vi "Read Config.vi"() -> ()   [LabVIEW 2018]
uses:
  File Type.ctl
  Type Defs/Global Action.ctl
  GC-MSMSDevlopment/Type/_RT Configuration 2.ctl
  Type Defs/Configration.ctl
panel:
  out "Cal/Res":dbl[][](array[numeric])
  out "Configration":T1
  out "Error Out":errorcluster
  in  "Error In":errorcluster
  in  "Start Path":path
  in  "Display (T)":bool=TRUE
  in  "Config File Type":T3
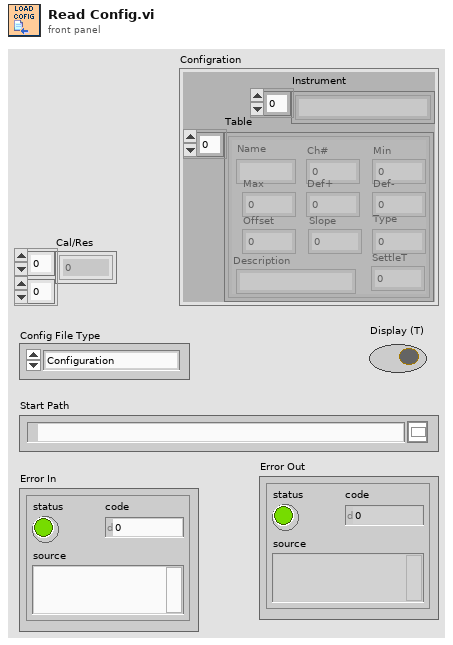
[diagram p1: front panel]
types:
  T1 = typedef "Configration.ctl" = cluster{"Table":T2[], "Instrument":string[]}
  T2 = typedef "_RT Configuration 2.ctl" = cluster{"Name":string, "Ch#":u8, "Min":dbl, "Max":dbl, "Def+":dbl, "Def-":dbl, "Offset":dbl, "Slope":dbl, "Type":u8, "Description":string, "SettleT":dbl}
  T3 = typedef "File Type.ctl" = enum16{"Configuration", "Old Configuration", "Calibration", "Resolution", "Diagnostic Method", "Old Method", "Acq Method", "Samp List"}
  T4 = typedef "Global Action.ctl" = enum16{"Write", "Read"}
  T5 = typedef "Global Configrations.ctl" = cluster{"Model Name":enum16{"QSight 110", "QSight 120", "QSight 210", "QSight 220", "QSight 410", "QSight 420", "IONICS 3Q 110", "IONICS 3Q 120", "IONICS 3Q 210", "IONICS 3Q 220", "IONICS 3Q 310", "IONICS 3Q 320", "Simulation (Single Source)", "Simulation (Dual Source)"}, "RunType":u16, "Acquisition State":enum16{"Ready", "Busy", "Waiting"}, "InstrState":enum16{"Initializing", "Mass Spectrometer is Off", "Starting Up", "Turning Power Off", "Going to Standby", "Roughing Pump Ready", "Turning Turbo Off", "Turbo Startup", "Turbopump Ready", "Checking Vacuum", "Going to Ready", "Ready", "Running", "Source Standby", "Lost Communication", "Shutting Down", "Fault", "24V Standby", "Go to 24V Standby", "Turbopump Ready-Waiting"}, "Run Mode":enum16{"MRM (Q1/Q2)", "Q1 Scan", "Q1 SRM", "Q2 Scan", "Q2 SRM", "Product Scan", "Precursor Scan", "Neutral Loss", "Neutral Gain"}, "Configration":T1, "TCP ID":refnum<k5>, "DT":bool, "Dead Time (nS)":i32, "Single Source":bool, "ADC Tables":T6[], "FW Udate":bool, "Simulator":bool}
  T6 = typedef "ADC Table.ctl" = cluster{"Name":string, "Ch#":u8, "Min":dbl, "Max":dbl, "Def+":dbl, "Def-":dbl, "Offset":dbl, "Slope":dbl, "Type":u8, "Description":string, "SettleT":dbl}
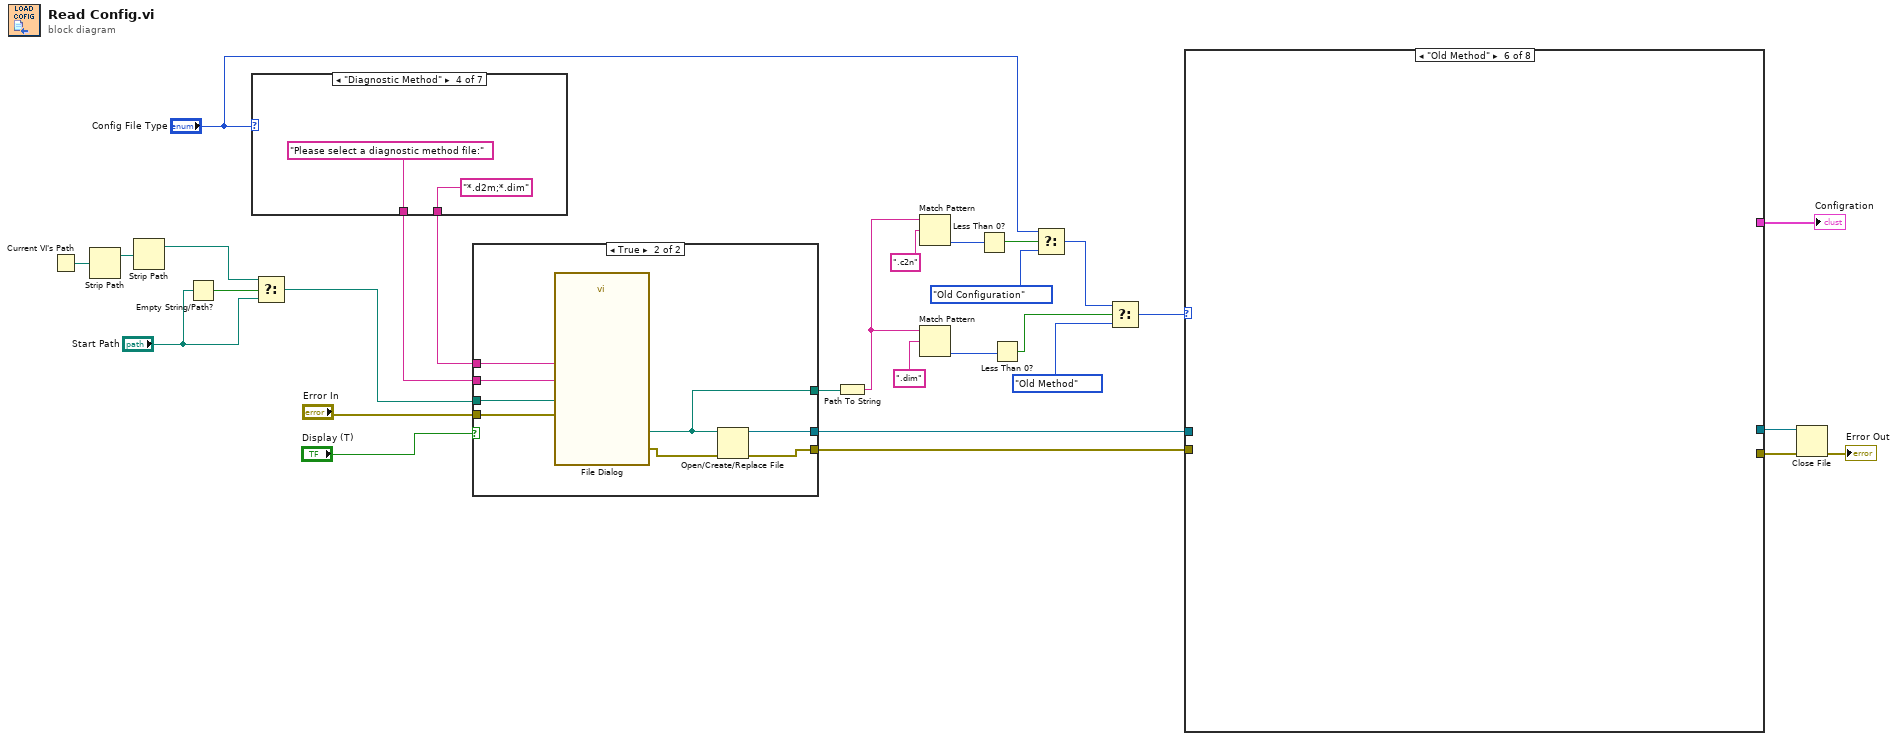
[diagram p0: block diagram]
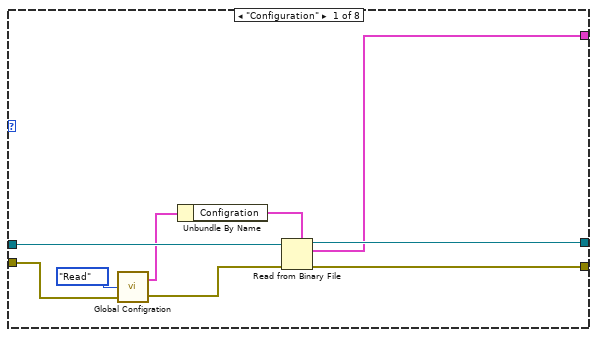
[diagram p2: hidden frame]
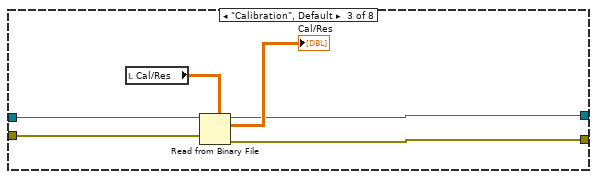
[diagram p4: hidden frame]
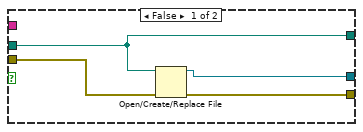
[diagram p9: hidden frame]
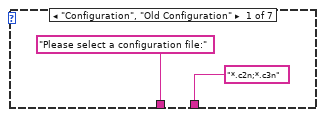
[diagram p10: hidden frame]
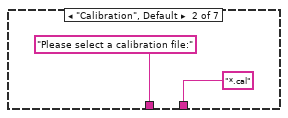
[diagram p11: hidden frame]
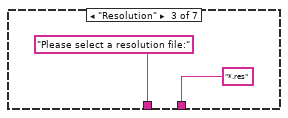
[diagram p12: hidden frame]
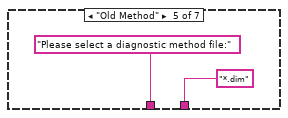
[diagram p13: hidden frame]
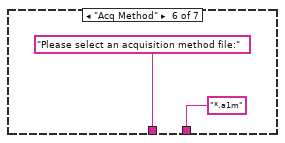
[diagram p14: hidden frame]
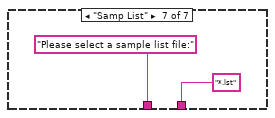
[diagram p15: hidden frame]
diagram:
  n1 = Current VI's Path() -> (path=w26:path)
  n2 = Strip Path(path=w26) -> (stripped path=w25:path)  [unwired: 1 out]
  n3 = Strip Path(path=w25) -> (stripped path=w23:path)  [unwired: 1 out]
  n4 = Empty String/Path?(string/path="Start Path") -> (empty?=w22:bool)
  n5 = case shown="\"Diagnostic Method\"" "Config File Type" {
    tunnel: ["*.c2n;*.c3n" ("pattern (*.cfg)") "*.cal" ("pattern (*.cfg)") "*.res" ("pattern (*.cfg)") "*.d2m;*.dim" ("pattern (*.cfg)") "*.dim" ("pattern (*.cfg)") "*.a1m" ("pattern (*.cfg)") "*.lst" ("pattern (*.cfg)")] -> w28
    tunnel: ["Please select a configuration file:" ("prompt") "Please select a calibration file:" ("prompt") "Please select a resolution file:" ("prompt") "Please select a diagnostic method file:" ("prompt") "Please select a diagnostic method file:" ("prompt") "Please select an acquisition method file:" ("prompt") "Please select a sample list file:" ("prompt")] -> w27
    frame "Configuration", "Old Configuration" {
    }
    frame "Calibration", Default {
    }
    frame "Resolution" {
    }
    frame "Diagnostic Method" {
    }
    frame "Old Method" {
    }
    frame "Acq Method" {
    }
    frame "Samp List" {
    }
  }
  n6 = Select(t=w23, s=w22, f="Start Path") -> (s? t:f=w24:path)
  n7 = case shown="True" "Display (T)" {
    tunnel: w28 -> [_ w55]
    tunnel: w27 -> [_ w54]
    tunnel: w24 -> [w44 w53]
    tunnel: "Error In" -> [w47 w52]
    tunnel: [w45 w50] -> w6
    tunnel: [w46 w49] -> w5
    tunnel: [w44 w48] -> w19
    frame False {
      n8 = Open/Create/Replace File(file path (use dialog)=w44, error in=w47) -> (refnum out=w45:refnum<file>, error out=w46:errorcluster)  [unwired: 4 in, 1 out]
    }
    frame True {
      n9 = call "File Dialog"("start path"=w53, "prompt"=w54, "error in"=w52, "pattern (all files)"=w55) -> ("selected path"=w48:path, "error out"=w51:errorcluster)  [unwired: 8 in, 2 out]
      n10 = Open/Create/Replace File(file path (use dialog)=w48, error in=w51) -> (refnum out=w50:refnum<file>, error out=w49:errorcluster)  [unwired: 4 in, 1 out]
    }
  }
  n11 = Path To String(path=w19) -> (string=w12:string)
  n12 = Match Pattern(string=w12, regular expression=".c2n") -> (offset past match=w13:i32)  [unwired: 4 out]
  n13 = Match Pattern(string=w12, regular expression=".dim") -> (offset past match=w17:i32)  [unwired: 4 out]
  n14 = Less Than 0?(x=w13) -> (x < 0?=w11:bool)
  n15 = Less Than 0?(x=w17) -> (x < 0?=w16:bool)
  n16 = Select(t="Config File Type", s=w11, f=File_Type."Old Configuration" ("Config File Type")) -> (s? t:f=w14:T3)
  n17 = Select(t=w14, s=w16, f=File_Type."Old Method" ("Config File Type")) -> (s? t:f=w7:T3)
  n18 = case shown="\"Old Method\"" w7 {
    tunnel: w6 -> [w64 _ w69 _ _ _ _ _]
    tunnel: w5 -> [w61 _ w70 _ _ _ _ _]
    tunnel: [w63 _ w65 _ _ _ _ _] -> w4
    tunnel: [w57 _ w66 _ _ _ _ _] -> w2
    tunnel: [w56 _ _ _ _ _ _ _] -> w1
    frame "Configuration" {
      n19 = call "Global Configration.vi"("Error In"=w61, "Action"=Global_Action."Read") -> ("Error Out"=w62:errorcluster, "Parameters Out"=w58:T5)  [unwired: 1 in]
      n20 = Unbundle By Name(w58) -> ("Configration"=w59:T1)
      n21 = Read from Binary File(5:w59, 8:w62, 11:w64) -> (0:w57:errorcluster, 2:w56:T1, 3:w63:refnum<file>)  [unwired: 4 out]
    }
    frame "Old Configuration" {
    }
    frame "Calibration", Default {
      n22 = local read "Cal/Res"() -> (w68:dbl[][])
      n23 = Read from Binary File(5:w68, 8:w70, 11:w69) -> (0:w66:errorcluster, 2:→"Cal/Res":dbl[][], 3:w65:refnum<file>)  [unwired: 3 in, 1 out]
    }
    frame "Resolution" {
    }
    frame "Diagnostic Method" {
    }
    frame "Old Method" {
    }
    frame "Acq Method" {
    }
    frame "Samp List" {
    }
  }
  "Configration" <- w1
  n24 = Close File(refnum=w4, error in=w2) -> (error out=→"Error Out":errorcluster)  [unwired: 1 out]
